vi "Select Ball By Confidence.vi"(10 "Array":T1[](array[typedef]) {"robots_blue"."height" format="%+4.3f"; "robots_blue"."pixel_y" format="%+4.3f"; "robots_blue"."pixel_x" format="%+4.3f"; "robots_blue"."orientation" format="%+4.3f"; "robots_blue"."y" format="%+4.3f"; "robots_blue"."confidence" format="%4.3f"; "robots_blue"."x" format="%+4.3f"; "robots_yellow"."height" format="%+4.3f"; "robots_yellow"."pixel_y" format="%+4.3f"; "robots_yellow"."pixel_x" format="%+4.3f"; "robots_yellow"."orientation" format="%+4.3f"; "robots_yellow"."y" format="%+4.3f"; "robots_yellow"."confidence" format="%4.3f"; "robots_yellow"."x" format="%+4.3f"}, 11 "balls":T4[](array[typedef])) -> (3 "balls out":T4[](array[typedef]))   [LabVIEW 2018]
uses:
  Controls/SSL Detection Ball.ctl
  <vilib>/Analysis/Matrix/Datatypes/RealMatrix.ctl
  Controls/SSL Detection Frame.ctl
  Controls/SSL Detection Robot.ctl
  <vilib>/Analysis/Matrix/NI_Matrix.lvlib
panel:
  in  "Boolean":bool
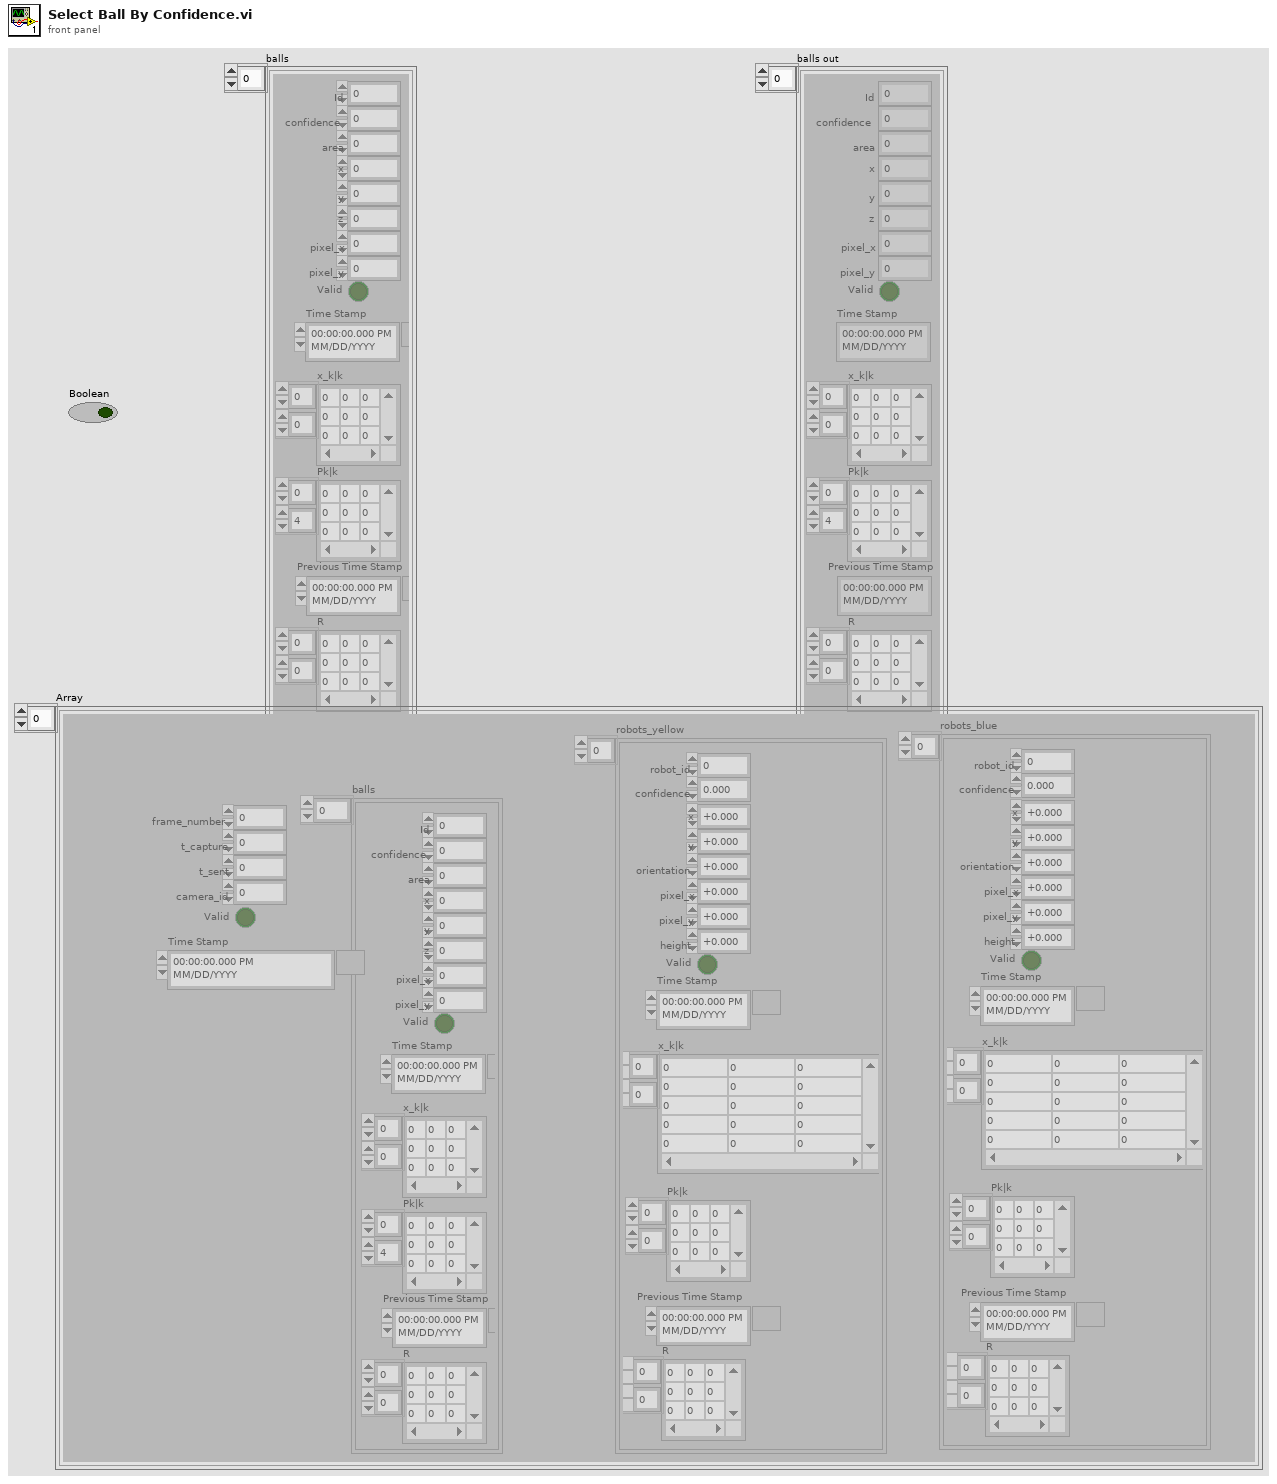
[diagram p1: front panel]
types:
  T1 = typedef "SSL Detection Frame.ctl" = cluster{"frame_number":u32, "t_capture":dbl, "t_sent":dbl, "camera_id":u32, "robots_yellow":T2[], "robots_blue":T2[], "balls":T4[], "Valid":bool, "Time Stamp":timestamp}
  T2 = typedef "SSL Detection Robot.ctl" = cluster{"x":sgl, "robot_id":u32, "confidence":sgl, "y":sgl, "orientation":sgl, "pixel_x":sgl, "pixel_y":sgl, "height":sgl, "Valid":bool, "Time Stamp":timestamp, "x_k|k":T3, "Pk|k":T3, "Previous Time Stamp":timestamp, "R":T3}
  T3 = typedef "NI_Matrix.lvlib/RealMatrix.ctl" = dbl[][]
  T4 = typedef "SSL Detection Ball.ctl" = cluster{"x":sgl, "area":u32, "confidence":sgl, "y":sgl, "z":sgl, "pixel_x":sgl, "pixel_y":sgl, "Valid":bool, "Time Stamp":timestamp, "x_k|k":T3, "Pk|k":T3, "Id":u32, "Previous Time Stamp":timestamp, "R":T3}
  T5 = cluster{"confidence":dbl, i32, "x":sgl, "y":sgl}[]
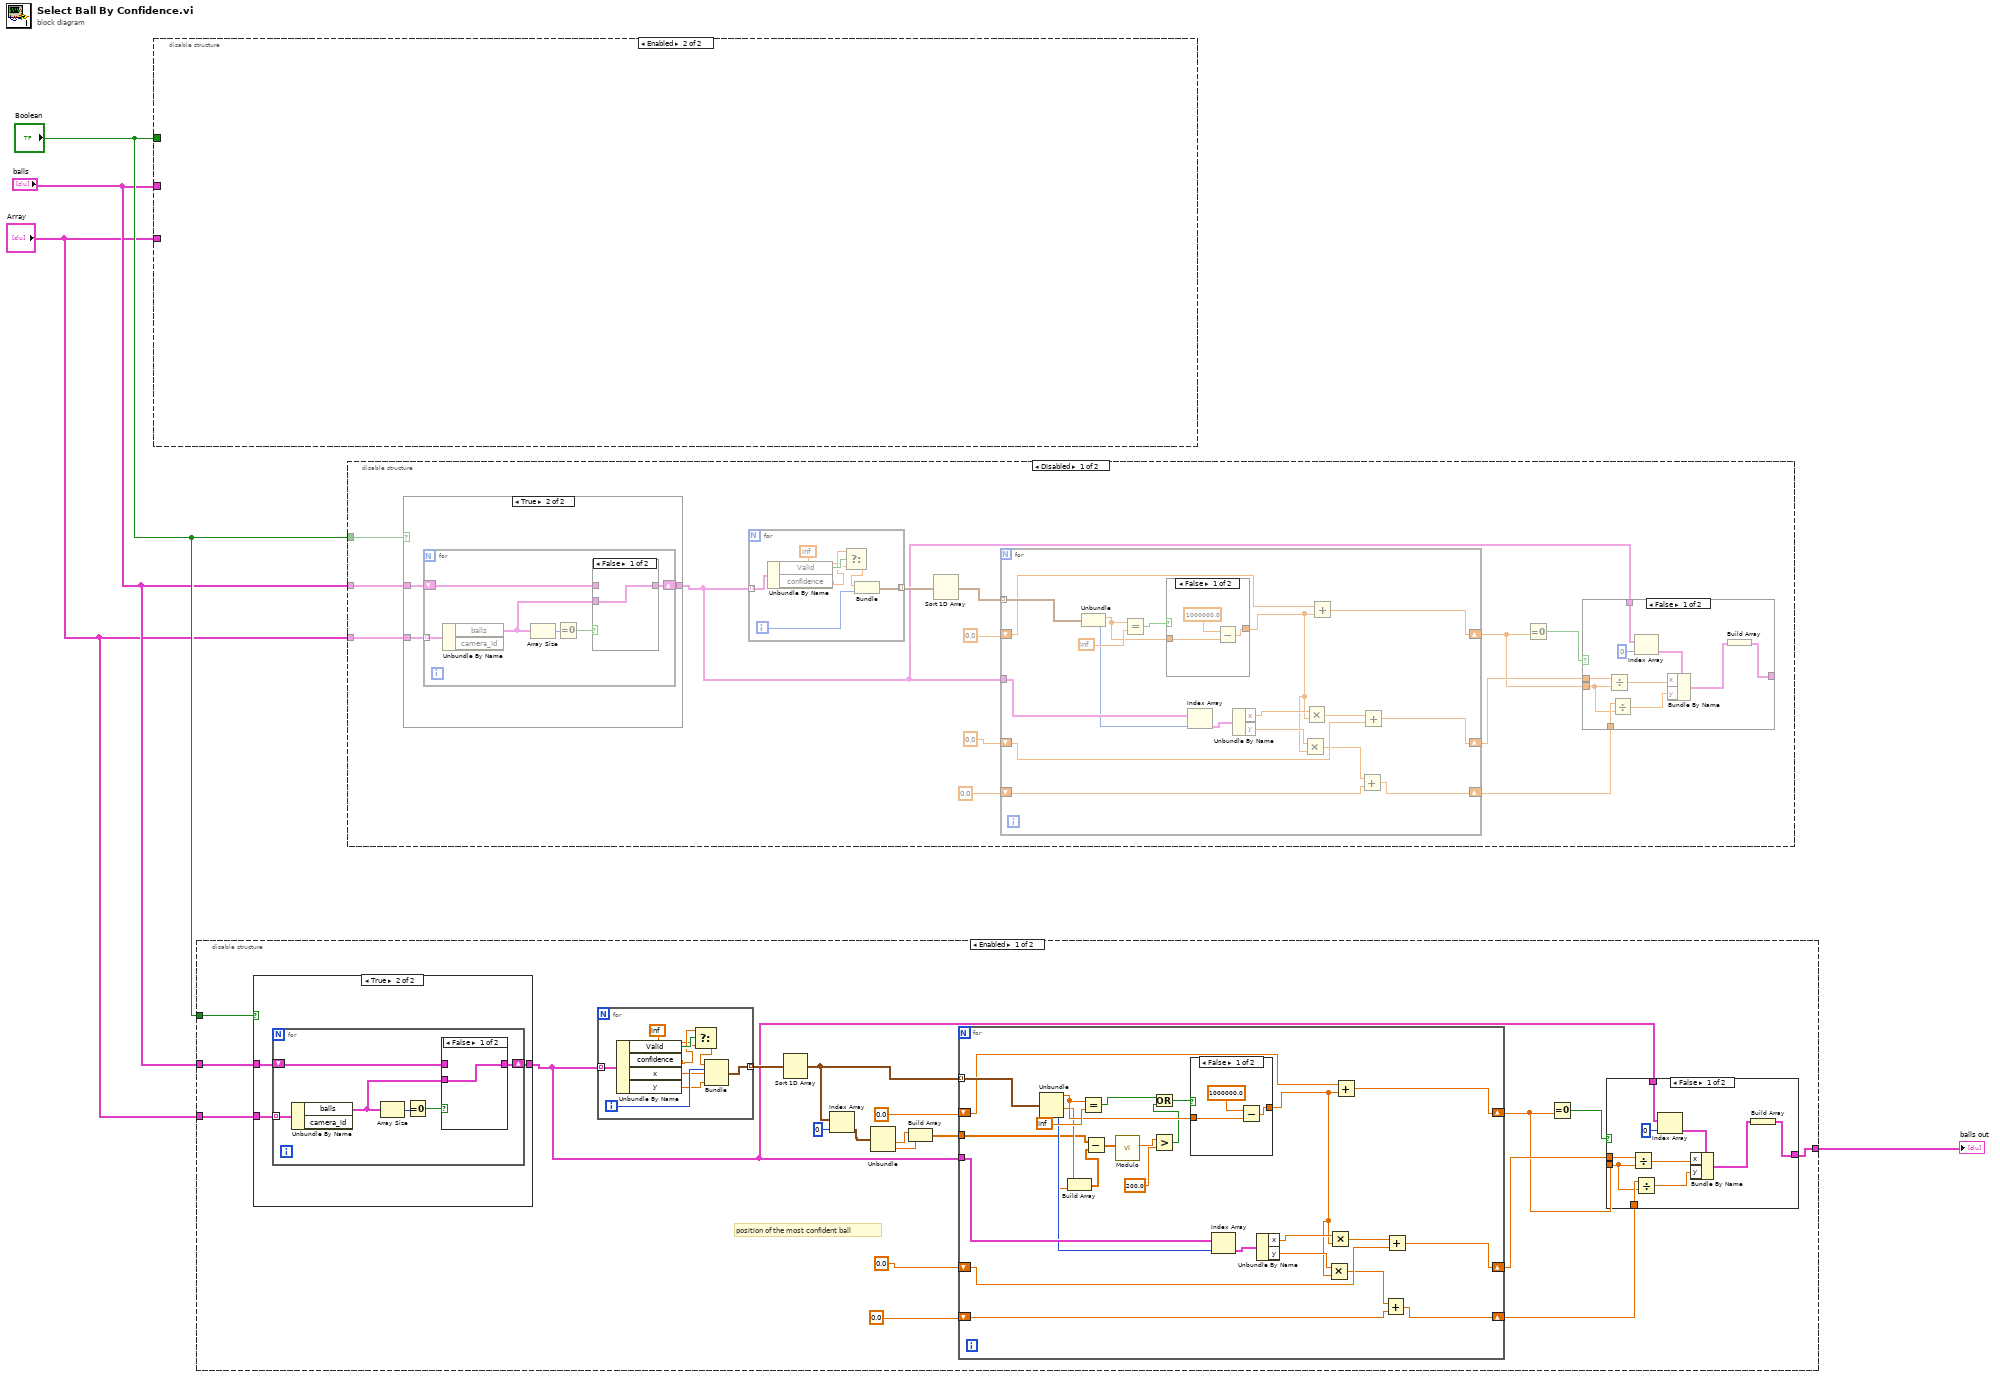
[diagram p0: block diagram]
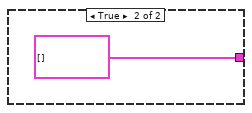
[diagram p2: hidden frame]
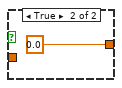
[diagram p3: hidden frame]
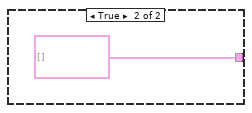
[diagram p7: hidden frame]
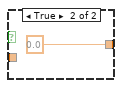
[diagram p8: hidden frame]
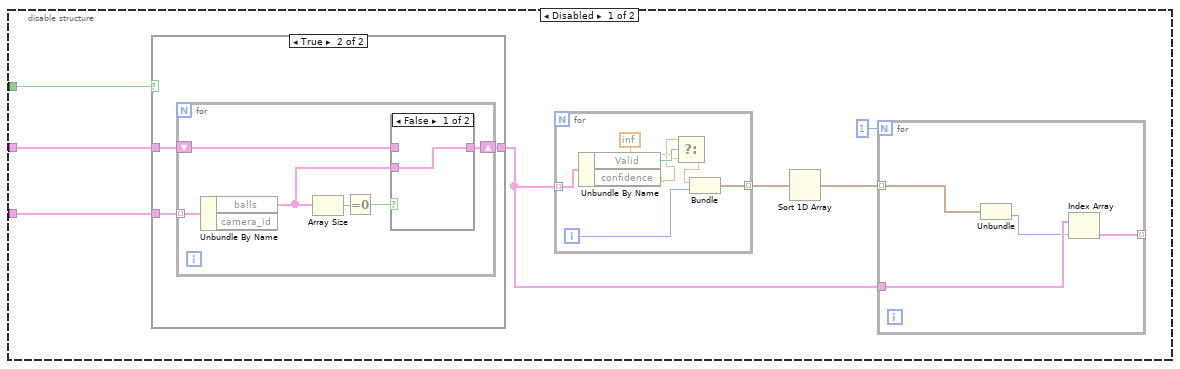
[diagram p12: hidden frame]
diagram:
  n1 = disable-structure shown="Enabled" {
    disable-tunnel: "Array" -> [w8 _]
    disable-tunnel: "balls" -> [w6 _]
    disable-tunnel: "Boolean" -> [w5 _]
    frame Disabled {
      n2 = case shown="True" w5 {
        tunnel: w8 -> [_ w15]
        tunnel: [w12 w14] -> w7
        tunnel: w6 -> [w12 w13]
        frame False {
        }
        frame True {
          n3 = for {
            tunnel: w15 -> [w21] mode=indexing
            shift-right: [w18] -> w14
            shift-left: w13 -> [w16]
            n4 = Unbundle By Name(w21) -> ("balls"=w17:T4[])  [unwired: 1 out]
            n5 = Array Size(array=w17) -> (size(s)=w20:i32)
            n6 = Equal To 0?(x=w20) -> (x = 0?=w19:bool)
            n7 = case shown="False" w19 {
              tunnel: [w22 w23] -> w18
              tunnel: w17 -> [w22 _]
              tunnel: w16 -> [_ w23]
              frame False {
              }
              frame True {
              }
            }
          }
        }
      }
      n8 = for {
        tunnel: w7 -> [w34] mode=indexing
        tunnel: [w33] -> w11 mode=indexing
        i -> [w32]
        n9 = Unbundle By Name(w34) -> ("Valid"=w31:bool, "confidence"=w30:sgl)
        n10 = Select(t=w30, s=w31, f=inf) -> (s? t:f=w29:dbl)
        n11 = Bundle("confidence"=w29, w32) -> (w33:cluster{"confidence":dbl, i32})  [unwired: 1 in]
      }
      n12 = Sort 1D Array(array=w11) -> (sorted array=w10:cluster{"confidence":dbl, i32}[])
      n13 = for {
        N: 1 -> [_]
        tunnel: w10 -> [w27] mode=indexing
        tunnel: w7 -> [w26]
        tunnel: [w24] -> _ mode=indexing
        n14 = Unbundle(w27) -> (w25:i32)  [unwired: 1 out]
        n15 = Index Array(array=w26, index=w25) -> (element=w24:T4)
      }
    }
    frame Enabled {
    }
  }
  n16 = disable-structure shown="Enabled" {
    disable-tunnel: "balls" -> [w53 _]
    disable-tunnel: "Array" -> [w52 _]
    disable-tunnel: "Boolean" -> [w51 _]
    disable-tunnel: [w41 _] -> w1
    frame Enabled {
      # "position of the most confident ball"
      n17 = case shown="True" w51 {
        tunnel: w52 -> [_ w108]
        tunnel: [w105 w107] -> w45
        tunnel: w53 -> [w105 w106]
        frame False {
        }
        frame True {
          n18 = for {
            tunnel: w108 -> [w114] mode=indexing
            shift-right: [w111] -> w107
            shift-left: w106 -> [w109]
            n19 = Unbundle By Name(w114) -> ("balls"=w110:T4[])  [unwired: 1 out]
            n20 = Array Size(array=w110) -> (size(s)=w113:i32)
            n21 = Equal To 0?(x=w113) -> (x = 0?=w112:bool)
            n22 = case shown="False" w112 {
              tunnel: [w115 w116] -> w111
              tunnel: w110 -> [w115 _]
              tunnel: w109 -> [_ w116]
              frame False {
              }
              frame True {
              }
            }
          }
        }
      }
      n23 = for {
        tunnel: w45 -> [w104] mode=indexing
        tunnel: [w103] -> w50 mode=indexing
        i -> [w102]
        n24 = Unbundle By Name(w104) -> ("Valid"=w101:bool, "confidence"=w100:sgl, "x"=w97:sgl, "y"=w96:sgl)
        n25 = Select(t=w100, s=w101, f=inf) -> (s? t:f=w99:dbl)
        n26 = Bundle("confidence"=w99, w102, "x"=w97, "y"=w96) -> (w103:cluster{"confidence":dbl, i32, "x":sgl, "y":sgl})  [unwired: 1 in]
      }
      n27 = Sort 1D Array(array=w50) -> (sorted array=w40:T5)
      n28 = Index Array(array=w40, index=0) -> (element=w38:cluster{"confidence":dbl, i32, "x":sgl, "y":sgl})
      n29 = Unbundle(w38) -> ("x"=w37:sgl, "y"=w36:sgl)  [unwired: 2 out]
      n30 = Build Array(w37, w36) -> (w35:sgl[])
      n31 = for {
        tunnel: w40 -> [w91] mode=indexing
        tunnel: w45 -> [w88]
        shift-right: [w84] -> w43
        shift-left: 0.0 -> [w85]
        shift-right: [w78] -> w44
        shift-left: 0.0 -> [w79]
        shift-right: [w75] -> w42
        shift-left: 0.0 -> [w76]
        tunnel: w35 -> [w71]
        n32 = Unbundle(w91) -> ("confidence"=w89:dbl, w87:i32, "x"=w74:sgl, "y"=w73:sgl)
        n33 = Build Array(w74, w73) -> (w72:sgl[])
        n34 = Equal?(x=w89, y=inf) -> (x = y?=w67:bool)
        n35 = Subtract(x=w71, y=w72) -> (x-y=w70:sgl[])
        n36 = call "Modulo.vi"("2D vector"=w70) -> ("Modulo"=w69:dbl)  [unwired: 10 in]
        n37 = Greater?(x=w69, y=200.0) -> (0:w66:bool)
        n38 = Or(x=w67, y=w66) -> (x .or. y?=w65:bool)
        n39 = case shown="False" w65 {
          tunnel: [w92 0.0] -> w81
          tunnel: w89 -> [w93 _]
          frame False {
            n40 = Subtract(x=1000000.0, y=w93) -> (x-y=w92:dbl)
          }
          frame True {
          }
        }
        n41 = Index Array(array=w88, index=w87) -> (element=w86:T4)
        n42 = Unbundle By Name(w86) -> ("x"=w83:sgl, "y"=w82:sgl)
        n43 = Multiply(x=w82, y=w81) -> (x*y=w77:dbl)
        n44 = Multiply(x=w83, y=w81) -> (x*y=w80:dbl)
        n45 = Add(x=w85, y=w81) -> (x+y=w84:dbl)
        n46 = Add(x=w77, y=w76) -> (x+y=w75:dbl)
        n47 = Add(x=w80, y=w79) -> (x+y=w78:dbl)
      }
      n48 = Equal To 0?(x=w43) -> (x = 0?=w46:bool)
      n49 = case shown="False" w46 {
        tunnel: w45 -> [w63 _]
        tunnel: [w59 T4[] [] ("balls out")] -> w41
        tunnel: w44 -> [w58 _]
        tunnel: w43 -> [w55 _]
        tunnel: w42 -> [w56 _]
        frame False {
          n50 = Divide(x=w58, y=w55) -> (x/y=w57:dbl)
          n51 = Divide(x=w56, y=w55) -> (x/y=w54:dbl)
          n52 = Index Array(array=w63, index=0) -> (element=w61:T4)
          n53 = Bundle By Name(cluster=w61, "x"=w57, "y"=w54) -> (w60:T4)
          n54 = Build Array(w60) -> (w59:T4[])
        }
        frame True {
        }
      }
    }
    frame Disabled {
    }
  }
  "balls out" <- w1
  n55 = disable-structure shown="Disabled" {
    disable-tunnel: "balls" -> [w129 _]
    disable-tunnel: "Array" -> [w128 _]
    disable-tunnel: "Boolean" -> [w127 _]
    frame Disabled {
      n56 = case shown="True" w127 {
        tunnel: w128 -> [_ w173]
        tunnel: [w170 w172] -> w120
        tunnel: w129 -> [w170 w171]
        frame False {
        }
        frame True {
          n57 = for {
            tunnel: w173 -> [w179] mode=indexing
            shift-right: [w176] -> w172
            shift-left: w171 -> [w174]
            n58 = Unbundle By Name(w179) -> ("balls"=w175:T4[])  [unwired: 1 out]
            n59 = Array Size(array=w175) -> (size(s)=w178:i32)
            n60 = Equal To 0?(x=w178) -> (x = 0?=w177:bool)
            n61 = case shown="False" w177 {
              tunnel: [w180 w181] -> w176
              tunnel: w175 -> [w180 _]
              tunnel: w174 -> [_ w181]
              frame False {
              }
              frame True {
              }
            }
          }
        }
      }
      n62 = for {
        tunnel: w120 -> [w169] mode=indexing
        tunnel: [w168] -> w126 mode=indexing
        i -> [w167]
        n63 = Unbundle By Name(w169) -> ("Valid"=w166:bool, "confidence"=w165:sgl)
        n64 = Select(t=w165, s=w166, f=inf) -> (s? t:f=w164:dbl)
        n65 = Bundle("confidence"=w164, w167) -> (w168:cluster{"confidence":dbl, i32})  [unwired: 1 in]
      }
      n66 = Sort 1D Array(array=w126) -> (sorted array=w125:cluster{"confidence":dbl, i32}[])
      n67 = for {
        tunnel: w125 -> [w158] mode=indexing
        tunnel: w120 -> [w154]
        shift-right: [w150] -> w118
        shift-left: 0.0 -> [w151]
        shift-right: [w144] -> w119
        shift-left: 0.0 -> [w145]
        shift-right: [w141] -> w117
        shift-left: 0.0 -> [w142]
        n68 = Unbundle(w158) -> ("confidence"=w155:dbl, w153:i32)
        n69 = Equal?(x=w155, y=inf) -> (x = y?=w156:bool)
        n70 = case shown="False" w156 {
          tunnel: [w159 0.0] -> w147
          tunnel: w155 -> [w160 _]
          frame False {
            n71 = Subtract(x=1000000.0, y=w160) -> (x-y=w159:dbl)
          }
          frame True {
          }
        }
        n72 = Index Array(array=w154, index=w153) -> (element=w152:T4)
        n73 = Unbundle By Name(w152) -> ("x"=w149:sgl, "y"=w148:sgl)
        n74 = Multiply(x=w148, y=w147) -> (x*y=w143:dbl)
        n75 = Multiply(x=w149, y=w147) -> (x*y=w146:dbl)
        n76 = Add(x=w151, y=w147) -> (x+y=w150:dbl)
        n77 = Add(x=w143, y=w142) -> (x+y=w141:dbl)
        n78 = Add(x=w146, y=w145) -> (x+y=w144:dbl)
      }
      n79 = Equal To 0?(x=w118) -> (x = 0?=w121:bool)
      n80 = case shown="False" w121 {
        tunnel: w120 -> [w139 _]
        tunnel: [w135 T4[] [] ("balls out")] -> _
        tunnel: w119 -> [w134 _]
        tunnel: w118 -> [w131 _]
        tunnel: w117 -> [w132 _]
        frame False {
          n81 = Divide(x=w134, y=w131) -> (x/y=w133:dbl)
          n82 = Divide(x=w132, y=w131) -> (x/y=w130:dbl)
          n83 = Index Array(array=w139, index=0) -> (element=w137:T4)
          n84 = Bundle By Name(cluster=w137, "x"=w133, "y"=w130) -> (w136:T4)
          n85 = Build Array(w136) -> (w135:T4[])
        }
        frame True {
        }
      }
    }
    frame Enabled {
    }
  }
